vi "Save Next 1D array.vi"(2 "ÆT":dbl format="%.2e", 3 "Data":dbl[](array[numeric]) format="%.2e", 4 "File Name":string="Test", 5 "Dir Path":path) -> (1 "New File Name":string)   [LabVIEW 2024]
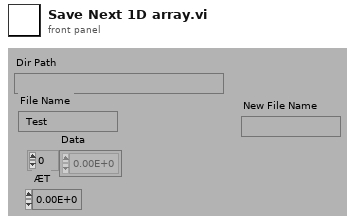
[diagram p1: front panel]
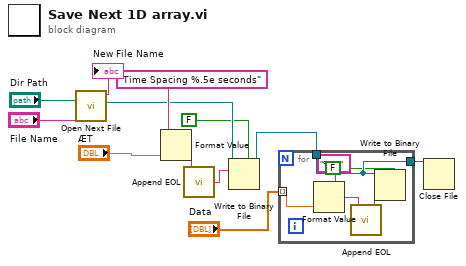
[diagram p0: block diagram]
diagram:
  n1 = call "Open Next File.vi"("Input File Pattern"="File Name", "Dir Path"="Dir Path") -> ("File Ref Num"=w3:refnum<file>, "Output File Name"=→"New File Name":string)  [unwired: 1 in, 2 out]
  n2 = Format Value(format string="Time Spacing %.5e seconds", value (0)="ÆT") -> (output string=w10:string)  [unwired: 1 in]
  n3 = call "Append EOL.vi"("INPUT STRING"=w10) -> ("OUTPUT STRING (PLUS End of Line)"=w9:string)
  n4 = Write to Binary File(file (use dialog)=w3, data=w9, 5:FALSE ("prepend array or string size? (T)")) -> (refnum out=w7:refnum<file>)  [unwired: 3 in, 2 out]
  n5 = for {
    tunnel: "Data" -> [w18] mode=indexing
    tunnel: w7 -> [w14]
    tunnel: [w14] -> w6
    n6 = Format Value(format string="%.8e", value (0)=w18) -> (output string=w16:string)  [unwired: 1 in]
    n7 = call "Append EOL.vi"("INPUT STRING"=w16) -> ("OUTPUT STRING (PLUS End of Line)"=w15:string)
    n8 = Write to Binary File(file (use dialog)=w14, data=w15, 5:FALSE ("prepend array or string size? (T)")) -> ()  [unwired: 3 in, 3 out]
  }
  n9 = Close File(refnum=w6) -> ()  [unwired: 1 in, 2 out]
